vi "Configure IQ.vi"(0 "VISA resource name":refnum<visa-resource-name>, 1 "Trigger Source (0: Internal)":u16(ring) items=["Internal", "External", "Manual"], 2 "Gain Balance(0 dB)":dbl, 3 "Q Channel Offset Value (0 V)":dbl, 5 "Center Frequency (0 Hz)":dbl, 7 "Symbol Rate (250 kSymbo/s)":dbl=250000.0, 9 "Amplitude (0.1414 Vrms)":dbl=0.1414, 11 "error in (no error)":errorcluster, 12 "I/Q Data (2ASK)":u16(ring) items=["2ASK", "4ASK", "8ASK", "BPSK", "QPSK", "8PSK", "DBPSK", "DQPSK", "D8PSK", "8QAM", "16QAM", "32QAM", "64QAM", "128QAM", "256QAM"], 13 "I Channel Offset Value (0 V)":dbl, 14 "Quadrature Skew (0 deg)":dbl) -> (4 "VISA resource name out":refnum<visa-resource-name>, 15 "error out":errorcluster)   [LabVIEW 2015, in "SDG X Series.lvlib"]
doc: "Configures I/Q modulation and parameters.\n\nNote:\nThis VI only supports SDG6000X series."
uses:
  <instrlib>/SDG X Series/SDG X Series.lvlib
panel:
  # "I/Q Adjustment"
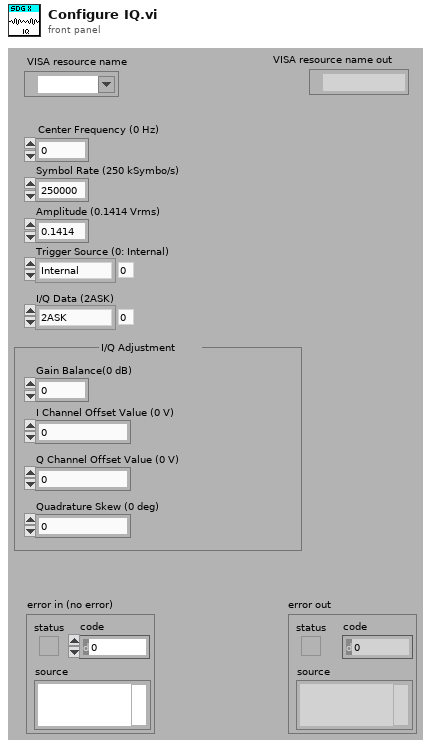
[diagram p1: front panel]
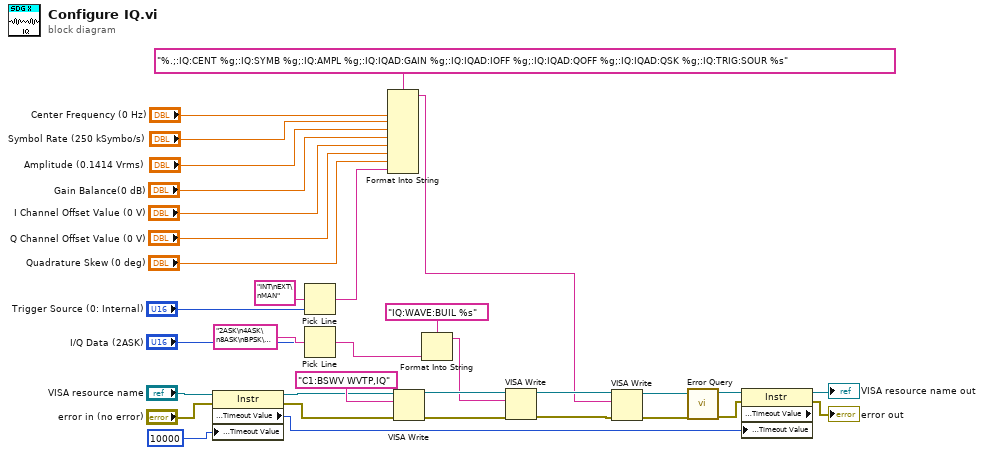
[diagram p0: block diagram]
diagram:
  n1 = property on="Property Node" class="Instr"(reference="VISA resource name", error in="error in (no error)", "General Settings:Timeout Value"=u32 10000) -> (reference out=w7:refnum<visa-resource-name>, error out=w10:errorcluster, "General Settings:Timeout Value"=w2:u32)
  n2 = Pick Line(multi-line string="INT\nEXT\nMAN" ("多行字符串"), line index="Trigger Source (0: Internal)") -> (output string=w14:string)  [unwired: 1 in]
  n3 = Pick Line(multi-line string="2ASK\n4ASK\n8ASK\nBPSK\nQPSK\n8PSK\nDBPSK\nDQPSK\nD8PSK\n8QAM\n16QAM\n32QAM\n64QAM\n128QAM\n256QAM" ("多行字符串"), line index="I/Q Data (2ASK)") -> (output string=w28:string)  [unwired: 1 in]
  n4 = Format Into String(format string="%.;:IQ:CENT %g;:IQ:SYMB %g;:IQ:AMPL %g;:IQ:IQAD:GAIN %g;:IQ:IQAD:IOFF %g;:IQ:IQAD:QOFF %g;:IQ:IQAD:QSK %g;:IQ:TRIG:SOUR %s" ("格式字符串"), "Center Frequency (0 Hz)", "Symbol Rate (250 kSymbo/s)", "Amplitude (0.1414 Vrms)", "Gain Balance(0 dB)", "I Channel Offset Value (0 V)", "Q Channel Offset Value (0 V)", "Quadrature Skew (0 deg)", w14) -> (resulting string=w22:string)  [unwired: 2 in, 1 out]
  n5 = VISA Write(VISA resource name=w7, write buffer="C1:BSWV WVTP,IQ" ("写入缓冲区"), error in (no error)=w10) -> (VISA resource name out=w27:refnum<visa-resource-name>, error out=w26:errorcluster)  [unwired: 1 out]
  n6 = Format Into String(format string="IQ:WAVE:BUIL %s" ("初始字符串"), w28) -> (resulting string=w25:string)  [unwired: 2 in, 1 out]
  n7 = VISA Write(VISA resource name=w27, write buffer=w25, error in (no error)=w26) -> (VISA resource name out=w24:refnum<visa-resource-name>, error out=w23:errorcluster)  [unwired: 1 out]
  n8 = VISA Write(VISA resource name=w24, write buffer=w22, error in (no error)=w23) -> (VISA resource name out=w12:refnum<visa-resource-name>, error out=w11:errorcluster)  [unwired: 1 out]
  n9 = call <instrlib>:"Error Query.vi"("error in (no error)"=w11, "VISA resource name"=w12) -> ("error out"=w5:errorcluster, "VISA resource name out"=w6:refnum<visa-resource-name>)  [unwired: 6 in, 2 out]
  n10 = property on="Property Node" class="Instr" props=["General Settings:Timeout Value", "General Settings:Timeout Value"](reference=w6, error in=w5, "General Settings:Timeout Value"=w2) -> (reference out=→"VISA resource name out":refnum<visa-resource-name>, error out=→"error out":errorcluster)  [unwired: 1 out]
